vi "rs3 Burn Self Cal.vi"(7 "error in (no error)":errorcluster, 10 "device in":u64) -> (0 "error out":errorcluster, 1 "error":u64, 3 "Device out":u64, 4 "return":i32)   [LabVIEW 2017, in "libRealSense3.lvlib"]
doc: "Saves the self-calibration result permanently to flash memory.\n\nparam[in] device RealSense device\nparam[out] error if non-null, receives any error that occurs during this call, otherwise, errors are ignored\nreturn true if succeeded"
uses:
  libRealSense3.lvlib
  realsense2.dll
panel:
  # "RS3 Burn Tare Cal."
  # "(C) Intel Corp. 2019,  AGJ"
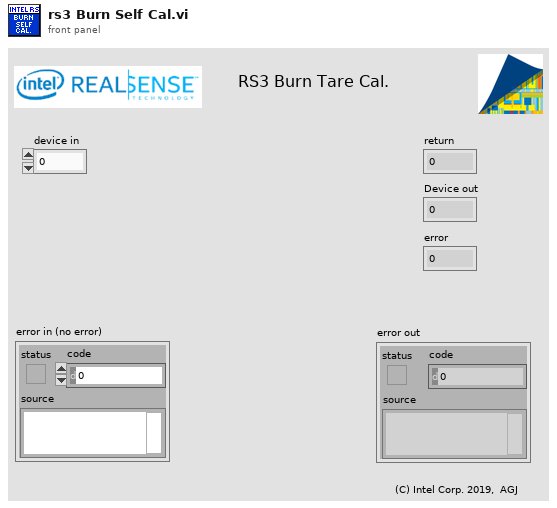
[diagram p1: front panel]
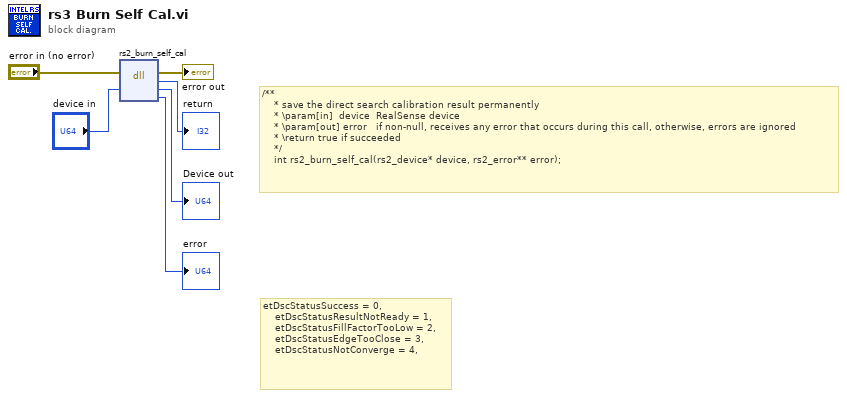
[diagram p0: block diagram]
diagram:
  # "/**\n    * save the direct search calibration result permanently\n    * \\param[in]  device  RealSense device\n    * \\param[out] error   if non-null, receives any error that occurs during this call, otherwise, errors are ignored\n    * \\return true if succeeded\n    */\n    int rs2_burn_self_cal(rs2_device* device, rs2_error** error);"
  # "etDscStatusSuccess = 0,\n    etDscStatusResultNotReady = 1,\n    etDscStatusFillFactorTooLow = 2,\n    etDscStatusEdgeTooClose = 3,\n    etDscStatusNotConverge = 4,"
  n1 = dll-call lib="C:/Users/agrunnet/Documents/libRealSense6/realsense2.dll" fn="rs2_burn_self_cal"(error in="error in (no error)", "device"="device in") -> (error out=→"error out":errorcluster, "result"=→"return":i32, "device"=→"Device out":u64, "error"=→"error":u64)  [unwired: 3 in, 1 out]
